vi "RegReadExt UnitTest.vi"() -> ()   [LabVIEW 2018]
uses:
  Downloads/MIPI RFFE API/Controls/RFFE Commands Type Def.ctl
  Downloads/MIPI RFFE API/Controls/Write Data Strict Type Def.ctl
  Command/RFFE Command.lvclass
  RegReadExt/RFFE RegReadExt Command.lvclass
  C:/Users/semoore/Projects/mipi-rffe-labview-oop/Command/RFFE Command.lvclass
panel:
  out "arrays same size?":bool
  out "data equal?":bool
  out "error in (no error) 2":errorcluster
  in  "error in (no error)":errorcluster
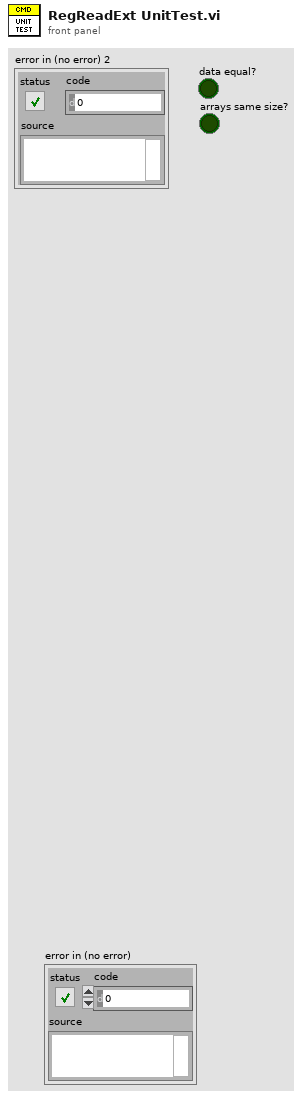
[diagram p1: front panel]
types:
  T1 = typedef "Write Data Strict Type Def.ctl" = cluster{"slave address":u8, "register address":u16, "register data (write)":u8[], "byte count":u8}
  T2 = typedef "RFFE Commands Type Def.ctl" = enum16{"Reg0Write", "RegWrite", "RegRead", "RegReadHR", "RegWriteExt", "RegReadExt", "RegReadExtHR", "RegWriteExtLong", "RegReadExtLong", "RegReadExtLongHR"}
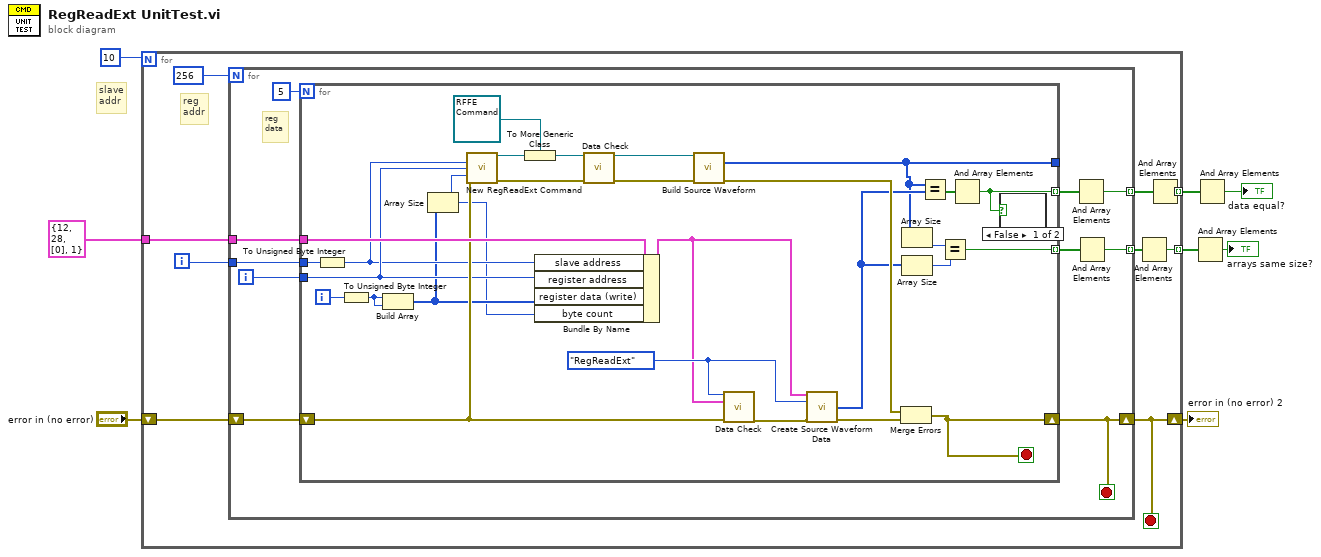
[diagram p0: block diagram]
diagram:
  # "slave\naddr"
  n1 = for {
    N: 10 -> [_]
    tunnel: T1 {"slave address"=12, "register address"=28, "register data (write)"=[0], "byte count"=1} ("Register Data") -> [w16]
    shift-right: [w13] -> w5
    shift-left: "error in (no error)" -> [w17]
    tunnel: [w11] -> w4 mode=indexing
    tunnel: [w9] -> w2 mode=indexing
    i -> [w15]
    stop <- w13 stop-if-true
    # "reg\naddr"
    n2 = for {
      N: 256 -> [_]
      tunnel: w16 -> [w26]
      tunnel: w15 -> [w23]
      shift-right: [w22] -> w13
      shift-left: w17 -> [w27]
      tunnel: [w20] -> w12 mode=indexing
      tunnel: [w18] -> w10 mode=indexing
      i -> [w24]
      stop <- w22 stop-if-true
      # "reg\ndata"
      n3 = for {
        N: 5 -> [_]
        tunnel: w26 -> [w53]
        tunnel: [w39] -> _
        tunnel: w24 -> [w33]
        tunnel: w23 -> [w42]
        shift-right: [w46] -> w22
        shift-left: w27 -> [w43]
        tunnel: [w36] -> w21 mode=indexing
        tunnel: [w31] -> w19 mode=indexing
        i -> [w41]
        stop <- w46 stop-if-true
        w55 = RFFE_Commands_Type_Def."RegReadExt" ("RFFE command")
        n4 = To Unsigned Byte Integer(number=w42) -> (unsigned 8bit integer=w32:u8)
        n5 = To Unsigned Byte Integer(number=w41) -> (unsigned 8bit integer=w30:u8)
        n6 = Build Array(w30, w30) -> (w29:u8[])
        n7 = Array Size(array=w29) -> (size(s)=w28:i32)
        n8 = call "New RegReadExt Command.vi"("Slave Address"=w32, "Register Address"=w33, "Byte Count"=w28, "error in (no error)"=w43) -> ("RFFE RegReadExt Command out"=w49:refnum<class "RFFE RegReadExt Command.lvclass">, "error out"=w50:errorcluster)  [unwired: 10 in]
        n9 = To More Generic Class(target class=refnum<class "RFFE Command.lvclass"> refnum ("RFFE Commands.lvlib:RFFE Command.lvclass"), reference=w49) -> (generic class reference=w35:refnum<class "RFFE Command.lvclass">)
        n10 = Bundle By Name(cluster=w53, "slave address"=w32, "register address"=w33, "register data (write)"=w29, "byte count"=w28) -> (w52:T1)
        n11 = call-dynamic "Data Check.vi"("RFFE Command in"=w35, "error in (no error)"=w50) -> ("RFFE Command out"=w48:refnum<class "RFFE Command.lvclass">, "error out"=w51:errorcluster)  [unwired: 12 in]
        n12 = call-dynamic "Build Source Waveform.vi"("RFFE Command in"=w48, "error in (no error)"=w51) -> ("Source Waveform"=w39:u32[], "error out"=w45:errorcluster)  [unwired: 11 in, 1 out]
        n13 = call "Data Check.vi"("RFFE command"=w55, "Register Data"=w52, "error in"=w43) -> ("error out"=w54:errorcluster)  [unwired: 12 in]
        n14 = call "Create Source Waveform Data.vi"("Register Data"=w52, "RFFE command"=w55, "error in"=w54) -> ("RFFEWrite source waveform data array"=w40:u32[], "error out"=w47:errorcluster)  [unwired: 10 in, 1 out]
        n15 = Merge Errors(w45, w47) -> (w46:errorcluster)
        n16 = Array Size(array=w39) -> (size(s)=w38:i32)
        n17 = Array Size(array=w40) -> (size(s)=w37:i32)
        n18 = Equal?(x=w39, y=w40) -> (x = y?=w44:bool[])
        n19 = Equal?(x=w38, y=w37) -> (x = y?=w31:bool)
        n20 = And Array Elements(Boolean array=w44) -> (logical AND=w36:bool)
        n21 = case shown="False" w36 {
          frame False {
          }
          frame True {
          }
        }
      }
      n22 = And Array Elements(Boolean array=w21) -> (logical AND=w20:bool)
      n23 = And Array Elements(Boolean array=w19) -> (logical AND=w18:bool)
    }
    n24 = And Array Elements(Boolean array=w10) -> (logical AND=w9:bool)
    n25 = And Array Elements(Boolean array=w12) -> (logical AND=w11:bool)
  }
  "error in (no error) 2" <- w5
  n26 = And Array Elements(Boolean array=w2) -> (logical AND=→"arrays same size?":bool)
  n27 = And Array Elements(Boolean array=w4) -> (logical AND=→"data equal?":bool)
